vi "REWORK_read_main_ini_file.vi"(8 "error_in":errorcluster) -> (0 "error_out":errorcluster, 1 "section_key_type_constant":string[][](array[string])=[["Paths", "References path", "path"], ["Paths", "Logs path", "path"], ["Paths", "User profiles", "path"], ["Connections", "UDP IP PC", "string"], ["Connections", "UDP port PC", "U16"], ["Connections", "UDP IP PLC", "string"], ["Connections", "UDP port PLC", "U16"], ["Connections", "TCP 1 IP PC", "string"], ["Connections", "TCP 1 port PC", "U16"], ["Connections", "TCP 2 IP PC", "string"], ["Connections", "TCP 2 port PC", "U16"], ["DAQ AI 1", "AI 1 Device number", "U8"], ["DAQ AI 1", "AI 1 Sample rate[S/s]", "double"], ["DAQ AI 1", "AI 1 Minimum value[V]", "double"], ["DAQ AI 1", "AI 1 Maximum value[V]", "double"], ["DAQ AI 1", "AI 1 Input terminal configuration", "ring"], ["DAQ AI 1", "AI 1 Sample mode", "ring"], ["DAQ AI 1", "AI 1 Temperature sensor resistance channel", "U8"], ["DAQ AI 1", "AI 1 Temperature sensor resistance range[V]", "double"], ["DAQ AI 1", "AI 1 Temperature sensor resistance nominal value[Ohm]", "double"], ["DAQ AI 1", "AI 1 Temperature sensor resistance offset[Ohm]", "double"], ["DAQ AI 1", "AI 1 Temperature sensor parallel resistor[Ohm]", "double"], ["DAQ AO 1", "AO 1 Device number", "U8"], ["DAQ AO 1", "AO 1 Output terminal configuration", "ring"], ["DAQ AO 1", "AO 1 Minimum value[V]", "double"], ["DAQ AO 1", "AO 1 Maximum value[V]", "double"], ["DAQ AO 1", "AO 1 Encoder power supply V program channel", "U8"], ["DAQ AO 1", "AO 1 Encoder power supply V program range min[V]", "double"], ["DAQ AO 1", "AO 1 Encoder power supply V program range max[V]", "double"], ["DAQ AO 1", "AO 1 Encoder power supply V program nominal value[V]", "double"], ["DAQ AO 1", "AO 1 Encoder power supply V program offset[V]", "double"], ["DAQ AO 1", "AO 1 Encoder power supply I program channel", "U8"], ["DAQ AO 1", "AO 1 Encoder power supply I program range min[V]", "double"], ["DAQ AO 1", "AO 1 Encoder power supply I program range max[V]", "double"], ["DAQ AO 1", "AO 1 Encoder power supply I program nominal value[A]", "double"], ["DAQ AO 1", "AO 1 Encoder power supply I program offset[V]", "double"], ["DAQ DI 1", "DI 1 Device number", "U8"], ["DAQ DI 1", "DI 1 Continuity Test Shield 1 port", "U8"], ["DAQ DI 1", "DI 1 Continuity Test Shield 1 line", "U8"], ["DAQ DI 1", "DI 1 Continuity Test Shield 2 port", "U8"], ["DAQ DI 1", "DI 1 Continuity Test Shield 2 line", "U8"], ["DAQ DO 1", "DO 1 Device number", "U8"], ["DAQ DO 1", "DO 1 Continuity Test Housing port", "U8"], ["DAQ DO 1", "DO 1 Continuity Test Housing line", "U8"], ["DAQ AI 2", "AI 2 Device number", "U8"], ["DAQ AI 2", "AI 2 Sample rate[S/s]", "double"], ["DAQ AI 2", "AI 2 Minimum value[V]", "double"], ["DAQ AI 2", "AI 2 Maximum value[V]", "double"], ["DAQ AI 2", "AI 2 Input terminal configuration", "ring"], ["DAQ AI 2", "AI 2 Sample mode", "ring"], ["DAQ AI 2", "AI 2 Embedded encoder A channel", "U8"], ["DAQ AI 2", "AI 2 Embedded encoder A range[V]", "double"], ["DAQ AI 2", "AI 2 Embedded encoder A nominal value[V]", "double"], ["DAQ AI 2", "AI 2 Embedded encoder A offset[V]", "double"], ["DAQ AI 2", "AI 2 Embedded encoder B channel", "U8"], ["DAQ AI 2", "AI 2 Embedded encoder B range[V]", "double"], ["DAQ AI 2", "AI 2 Embedded encoder B nominal value[V]", "double"], ["DAQ AI 2", "AI 2 Embedded encoder B offset[V]", "double"], ["DAQ AI 2", "AI 2 Embedded encoder current channel", "U8"], ["DAQ AI 2", "AI 2 Embedded encoder current range[V]", "double"], ["DAQ AI 2", "AI 2 Embedded encoder current nominal value[mA]", "double"], ["DAQ AI 2", "AI 2 Embedded encoder current offset[mA]", "double"], ["DAQ AI 2", "AI 2 Torque sensor channel", "U8"], ["DAQ AI 2", "AI 2 Torque sensor range[V]", "double"], ["DAQ AI 2", "AI 2 Torque sensor nominal value[Nm]", "double"], ["DAQ AI 2", "AI 2 Torque sensor offset[Nm]", "double"], ["DAQ AI 2", "AI 2 Motor power supply I monitor channel", "U8"], ["DAQ AI 2", "AI 2 Motor power supply I monitor range[V]", "double"], ["DAQ AI 2", "AI 2 Motor power supply I monitor nominal value[A]", "double"], ["DAQ AI 2", "AI 2 Motor power supply I monitor offset[A]", "double"], ["DAQ AI 2", "AI 2 Motor power supply V monitor channel", "U8"], ["DAQ AI 2", "AI 2 Motor power supply V monitor range[V]", "double"], ["DAQ AI 2", "AI 2 Motor power supply V monitor nominal value[V]", "double"], ["DAQ AI 2", "AI 2 Motor power supply V monitor offset[V]", "double"], ["DAQ AI 2", "AI 2 Encoder power supply I monitor channel", "U8"], ["DAQ AI 2", "AI 2 Encoder power supply I monitor range[V]", "double"], ["DAQ AI 2", "AI 2 Encoder power supply I monitor nominal value[A]", "double"], ["DAQ AI 2", "AI 2 Encoder power supply I monitor offset[A]", "double"], ["DAQ AI 2", "AI 2 Encoder power supply V monitor channel", "U8"], ["DAQ AI 2", "AI 2 Encoder power supply V monitor range[V]", "double"], ["DAQ AI 2", "AI 2 Encoder power supply V monitor nominal value[V]", "double"], ["DAQ AI 2", "AI 2 Encoder power supply V monitor offset[V]", "double"], ["DAQ CNT 2", "CNT 2 Device number", "U8"], ["DAQ CNT 2", "CNT 2 Counter number", "U8"], ["DAQ CNT 2", "CNT 2 Channel A PFI terminal", "U8"], ["DAQ CNT 2", "CNT 2 Channel B PFI terminal", "U8"], ["DAQ CNT 2", "CNT 2 Decoding type", "ring"], ["DAQ CNT 2", "CNT 2 Pulses per rotation", "I32"], ["DAQ AO 2", "AO 2 Device number", "U8"], ["DAQ AO 2", "AO 2 Output terminal configuration", "ring"], ["DAQ AO 2", "AO 2 Minimum value[V]", "double"], ["DAQ AO 2", "AO 2 Maximum value[V]", "double"], ["DAQ AO 2", "AO 2 Motor power supply V program channel", "U8"], ["DAQ AO 2", "AO 2 Motor power supply V program range min[V]", "double"], ["DAQ AO 2", "AO 2 Motor power supply V program range max[V]", "double"], ["DAQ AO 2", "AO 2 Motor power supply V program nominal value[V]", "double"], ["DAQ AO 2", "AO 2 Motor power supply V program offset[V]", "double"], ["DAQ AO 2", "AO 2 Motor power supply I program channel", "U8"], ["DAQ AO 2", "AO 2 Motor power supply I program range min[V]", "double"], ["DAQ AO 2", "AO 2 Motor power supply I program range max[V]", "double"], ["DAQ AO 2", "AO 2 Motor power supply I program nominal value[A]", "double"], ["DAQ AO 2", "AO 2 Motor power supply I program offset[A]", "double"], ["DAQ AO 2", "AO 2 Braker PS channel", "U8"], ["DAQ AO 2", "AO 2 Braker PS range min[V]", "double"], ["DAQ AO 2", "AO 2 Braker PS range max[V]", "double"], ["DAQ AO 2", "AO 2 Braker PS nominal value[A]", "double"], ["DAQ AO 2", "AO 2 Braker offset[Nm]", "double"], ["DAQ AO 2", "AO 2 Braker Torque at PS nominal value[Nm]", "double"], ["DAQ AO 2", "AO 2 Torque Input scaling a", "double"], ["DAQ AO 2", "AO 2 Torque Input scaling b", "double"], ["DAQ DI 2", "DI 2 Device number", "U8"], ["DAQ DI 2", "DI 2 Coupling OK port", "U8"], ["DAQ DI 2", "DI 2 Coupling OK line", "U8"], ["DAQ DO 2", "DO 2 Device number", "U8"], ["DAQ DO 2", "DO 2 Motor direction port", "U8"], ["DAQ DO 2", "DO 2 Motor direction line", "U8"]], 2 "config_info":T1, 3 "main_ini_file_out":T2={"SQL Driver"="", "SQL Server"="", "SQL Database"="", "SQL UID"="", "User table"="", "default language"="", "SCANNER COM port"=0, "SCANNER Baud rate"=0, "SCANNER Data bits"=0, "SCANNER Pairity"=enum."None", "SCANNER Stop bits"=10, "SCANNER Flow control"=0, "SCANNER Termination char"=0, "ST 140 name"="", "ST 140 listener IP"="", "ST 140 listener port"=0, "logout timeout [ms]"=0} {"SCANNER Flow control" items=["None"=0, "XON/XOFF"=1, "RTS/CTS"=2, "DTR/DSR"=4]; "SCANNER Stop bits" items=["1.0"=10, "1.5"=15, "2.0"=20]})   [LabVIEW 2019]
uses:
  typedef/REWORK_main_ini_file.ctl
  typedef/REWORK_config_info.ctl
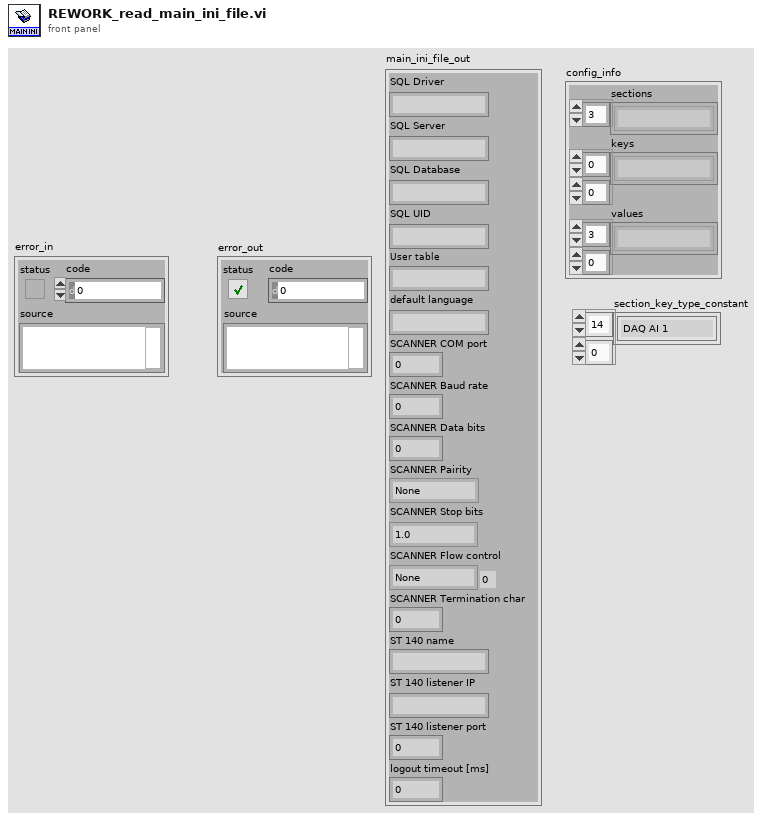
[diagram p1: front panel]
types:
  T1 = typedef "REWORK_config_info.ctl" = cluster{"sections":string[], "keys":string[][], "values":string[][]}
  T2 = typedef "REWORK_main_ini_file.ctl" = cluster{"SQL Driver":string, "SQL Server":string, "SQL Database":string, "SQL UID":string, "User table":string, "default language":string, "SCANNER COM port":u16, "SCANNER Baud rate":u32, "SCANNER Data bits":u16, "SCANNER Pairity":enum16{"None", "Odd", "Even", "Mark", "Space"}, "SCANNER Stop bits":u16, "SCANNER Flow control":u16, "SCANNER Termination char":u8, "ST 140 name":string, "ST 140 listener IP":string, "ST 140 listener port":u16, "logout timeout [ms]":i32}
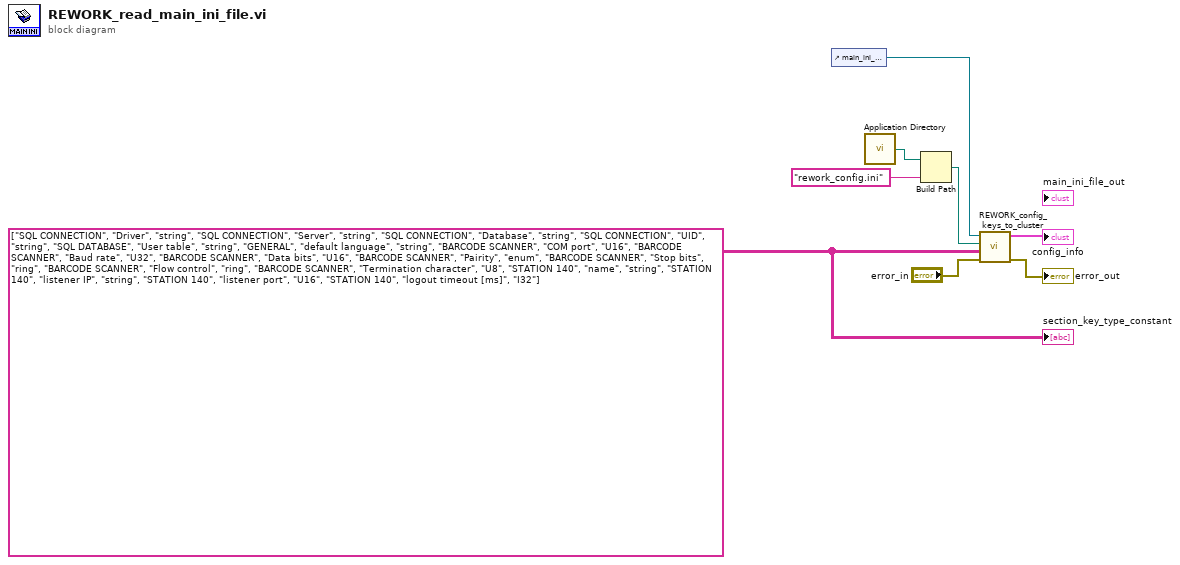
[diagram p0: block diagram]
diagram:
  w1 = string[][] [["SQL CONNECTION", "Driver", "string"], ["SQL CONNECTION", "Server", "string"], ["SQL CONNECTION", "Database", "string"], ["SQL CONNECTION", "UID", "string"], ["SQL DATABASE", "User table", "string"], ["GENERAL", "default language", "string"], ["BARCODE SCANNER", "COM port", "U16"], ["BARCODE SCANNER", "Baud rate", "U32"], ["BARCODE SCANNER", "Data bits", "U16"], ["BARCODE SCANNER", "Pairity", "enum"], ["BARCODE SCANNER", "Stop bits", "ring"], ["BARCODE SCANNER", "Flow control", "ring"], ["BARCODE SCANNER", "Termination character", "U8"], ["STATION 140", "name", "string"], ["STATION 140", "listener IP", "string"], ["STATION 140", "listener port", "U16"], ["STATION 140", "logout timeout [ms]", "I32"]]
  n1 = control-ref of="main_ini_file_out"() -> (w6:refnum<vi>)
  n2 = call <vilib>:"Application Directory.vi"() -> ("Application Directory"=w4:path)
  n3 = Build Path(base path=w4, name or relative path="rework_config.ini") -> (appended path=w2:path)
  n4 = call "REWORK_config_keys_to_cluster.vi"("error_in"="error_in", "section_key_type_table"=w1, "reference_ini_file_path"=w2, "config_cluster_ref"=w6) -> ("error_out"=→"error_out":errorcluster, "reference_info"=→"config_info":T1)  [unwired: 6 in]
  "section_key_type_constant" <- w1
